vi "Manipulatewave.vi"(8 "修改波形参数":T1, 9 "导入导出波形文件":T2, 10 "一炮最长运行时间点（ms)":dbl, 11 "预设波形数组":dbl[][](array[numeric])) -> (0 "波形数组":dbl[][](array[numeric]), 1 "波形解析正确":bool, 2 "XY Graph":cluster{"xi used":dbl[], "yi":dbl[]}(graph), 3 "插值后输出波形幅值":dbl[](array[numeric]))   [LabVIEW 2018]
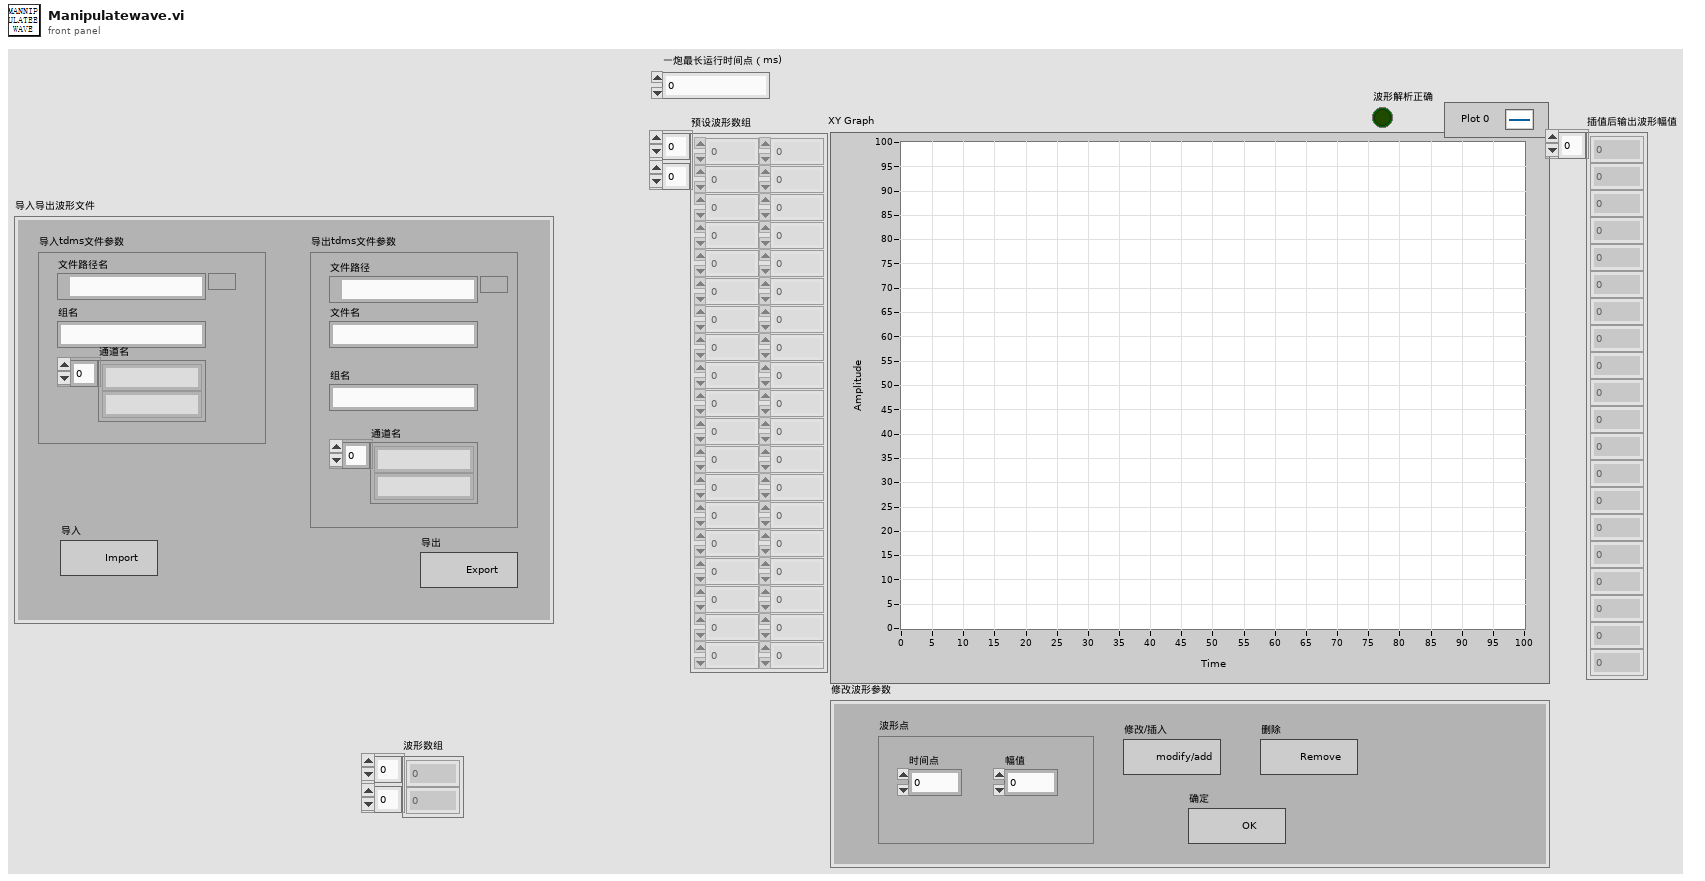
[diagram p1: front panel]
types:
  T1 = cluster{"波形点":cluster{"时间点":dbl, "幅值":dbl}, "修改/插入":bool, "删除":bool, "确定":bool}
  T2 = cluster{"导出tdms文件参数":cluster{"组名":string, "通道名":string[], "文件路径":path, "文件名":string}, "导入tdms文件参数":cluster{"文件路径名":path, "组名":string, "通道名":string[]}, "导入":bool, "导出":bool}
  T3 = cluster{"文件路径名":path, "组名":string, "通道名":string[]}
  T4 = cluster{"组名":string, "通道名":string[], "文件路径":path, "文件名":string}
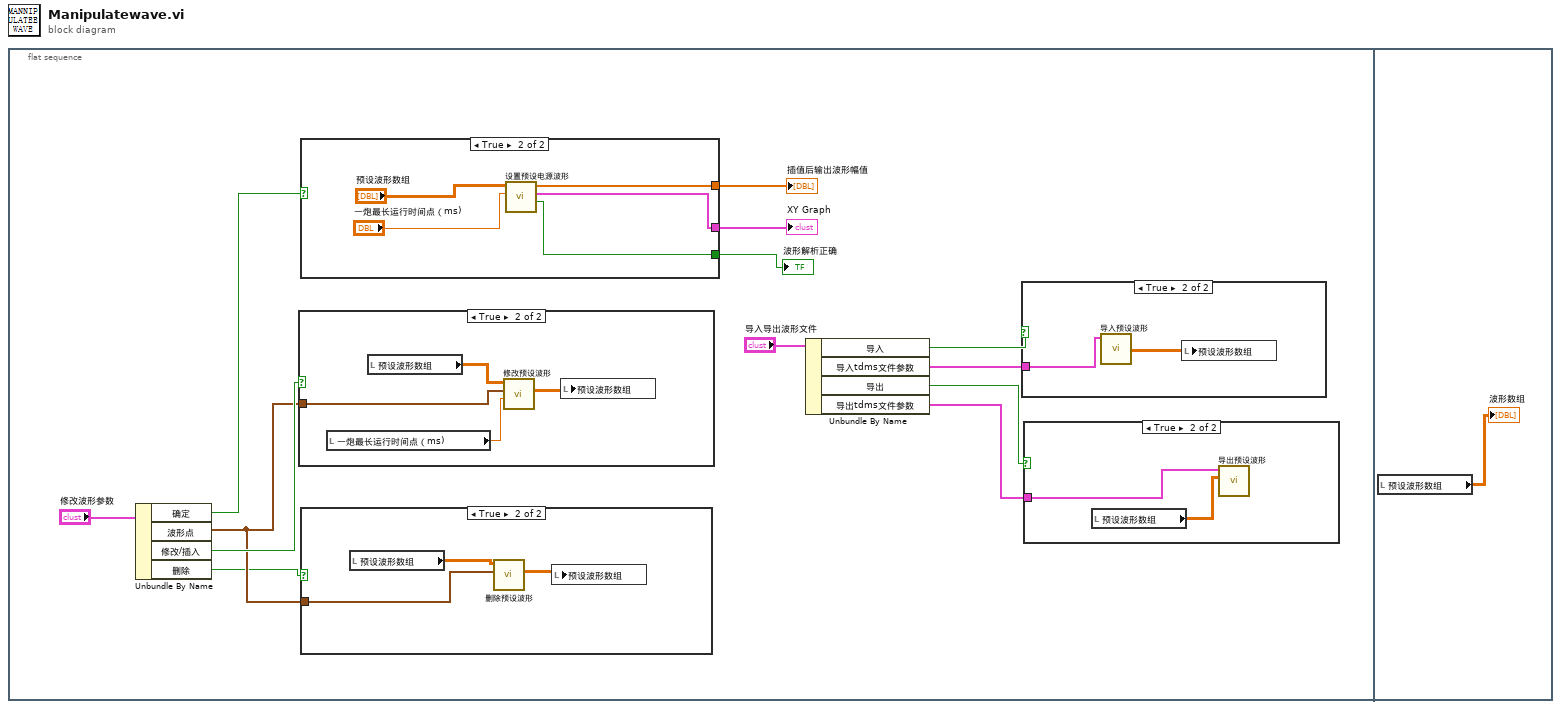
[diagram p0: block diagram]
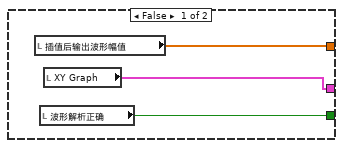
[diagram p4: hidden frame]
diagram:
  n1 = flat-sequence {
    frame #0 {
      n2 = Unbundle By Name("修改波形参数") -> ("确定"=w7:bool, "波形点"=w5:cluster{"时间点":dbl, "幅值":dbl}, "修改/插入"=w6:bool, "删除"=w4:bool)
      n3 = case shown="True" w6 {
        tunnel: w5 -> [_ w19]
        frame False {
        }
        frame True {
          n4 = local read "一炮最长运行时间点（ms)"() -> (w17:dbl)
          n5 = local read "预设波形数组"() -> (w20:dbl[][])
          n6 = call "修改预设波形.vi"("一炮最长运行时间"=w17, "波形点"=w19, "原预设波形"=w20) -> ("修改后波形"=w18:dbl[][])  [unwired: 8 in]
          n7 = local write "预设波形数组"(w18) -> ()
        }
      }
      n8 = case shown="True" w7 {
        tunnel: [w21 w26] -> w3
        tunnel: [w22 w25] -> w2
        tunnel: [w23 w24] -> w1
        frame False {
          n9 = local read "插值后输出波形幅值"() -> (w21:dbl[])
          n10 = local read "波形解析正确"() -> (w23:bool)
          n11 = local read "XY Graph"() -> (w22:cluster{"xi used":dbl[], "yi":dbl[]})
        }
        frame True {
          n12 = call "设置预设电源波形.vi"("一炮最长运行时间点（ms)"="一炮最长运行时间点（ms)", "预设波形数组"="预设波形数组") -> ("波形解析正确"=w24:bool, "XY Graph"=w25:cluster{"xi used":dbl[], "yi":dbl[]}, "插值后输出波形幅值"=w26:dbl[])  [unwired: 7 in]
        }
      }
      "插值后输出波形幅值" <- w3
      "XY Graph" <- w2
      "波形解析正确" <- w1
      n13 = case shown="True" w4 {
        tunnel: w5 -> [_ w15]
        frame False {
        }
        frame True {
          n14 = local read "预设波形数组"() -> (w16:dbl[][])
          n15 = call "删除预设波形.vi"("波形点"=w15, "原预设波形"=w16) -> ("删除后波形"=w14:dbl[][])  [unwired: 9 in]
          n16 = local write "预设波形数组"(w14) -> ()
        }
      }
      n17 = Unbundle By Name("导入导出波形文件") -> ("导入"=w12:bool, "导入tdms文件参数"=w11:T3, "导出"=w10:bool, "导出tdms文件参数"=w9:T4)
      n18 = case shown="True" w12 {
        tunnel: w11 -> [_ w32]
        frame False {
        }
        frame True {
          n19 = call "导入预设波形.vi"("导入tdms文件参数"=w32) -> ("预设波形数组"=w31:dbl[][])  [unwired: 10 in]
          n20 = local write "预设波形数组"(w31) -> ()
        }
      }
      n21 = case shown="True" w10 {
        tunnel: w9 -> [_ w30]
        frame False {
        }
        frame True {
          n22 = local read "预设波形数组"() -> (w29:dbl[][])
          n23 = call "导出预设波形.vi"("预设波形"=w29, "导出tdms文件参数"=w30) -> ()  [unwired: 10 in]
        }
      }
    }
    frame #1 {
      n24 = local read "预设波形数组"() -> (→"波形数组":dbl[][])
    }
  }
